vi "GEOM_CheckExtension.vi"(5 "extension to look":string="fpa", 9 "name in":string) -> (1 "rootname (no extension)":string, 2 "name out":string)   [LabVIEW 2016]
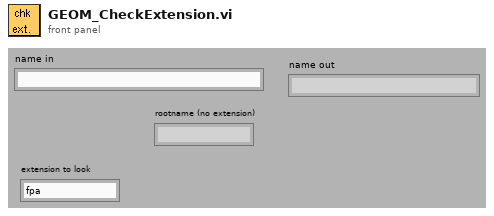
[diagram p1: front panel]
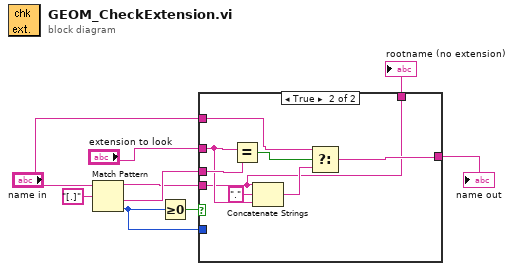
[diagram p0: block diagram]
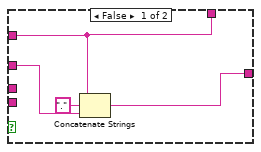
[diagram p2: hidden frame]
diagram:
  n1 = Match Pattern(string="name in", regular expression="[.]") -> (before substring=w2:string, after substring=w6:string, offset past match=w7:i32)  [unwired: 2 out]
  n2 = Greater Or Equal To 0?(x=w7) -> (x >= 0?=w8:bool)
  n3 = case shown="True" w8 {
    tunnel: w7 -> [_ _]
    tunnel: w6 -> [_ w21]
    tunnel: "extension to look" -> [w12 w16]
    tunnel: "name in" -> [w10 w19]
    tunnel: [w11 w18] -> w3
    tunnel: w2 -> [_ w14]
    tunnel: [w10 w14] -> w1
    frame False {
      n4 = Concatenate Strings(w10, "." ("string"), w12) -> (w11:string)
    }
    frame True {
      n5 = Equal?(x=w16, y=w21) -> (x = y?=w20:bool)
      n6 = Concatenate Strings(w14, "." ("string"), w16) -> (w15:string)
      n7 = Select(t=w19, s=w20, f=w15) -> (s? t:f=w18:string)
    }
  }
  "name out" <- w3
  "rootname (no extension)" <- w1
